vi "Read planetName.vi"(8 "error in (no error)":errorcluster, 11 "Planet in":refnum<class "Planet.lvclass">) -> (0 "error out":errorcluster, 2 "planetName":T1, 3 "Planet out":refnum<class "Planet.lvclass">)   [LabVIEW 2014, in "TCSDataDefinitions.lvlib" / "TCSCommand.lvlib" / "TargetConfiguration.lvlib" / "Target.lvlib" / "Planet.lvclass"]
uses:
  Planet.lvclass
  Enumerations/PlanetNameValues.ctl
  Planet.lvclass/Planet.ctl
  Target.lvlib
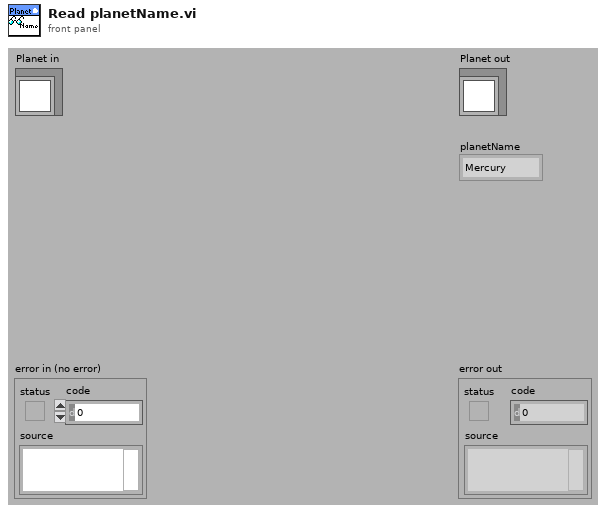
[diagram p1: front panel]
types:
  T1 = typedef "TCSDataDefinitions.lvlib/TCSCommand.lvlib/TargetConfiguration.lvlib/Target.lvlib/PlanetNameValues.ctl" = enum16{"Mercury", "Venus", "Moon", "Mars", "Jupiter", "Saturn", "Uranus", "Neptune", "Pluto"}
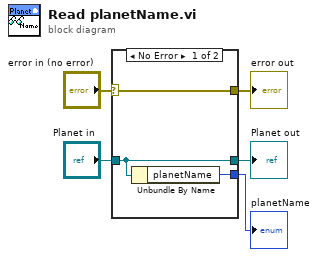
[diagram p0: block diagram]
diagram:
  n1 = case shown="No Error" "error in (no error)" {
    selector: "error in (no error)" -> [w8 w9]
    tunnel: [w8 w9] -> w4
    tunnel: [w7 w10] -> w2
    tunnel: "Planet in" -> [w7 w10]
    tunnel: [w6 _] -> w1
    frame No Error {
      n2 = Unbundle By Name(w7) -> ("planetName"=w6:T1)
    }
    frame Error {
    }
  }
  "error out" <- w4
  "Planet out" <- w2
  "planetName" <- w1
